vi "JPL Arm Control EX Autonomous.vi"(4 "Actual Angle":dbl, 5 "Arm Control":T1) -> (0 "Arm Status":T2, 3 "output":dbl)   [LabVIEW 2015]
panel:
  out "Arm Angle Chart":dbl(graph)
  out "PID Output Chart":dbl(graph)
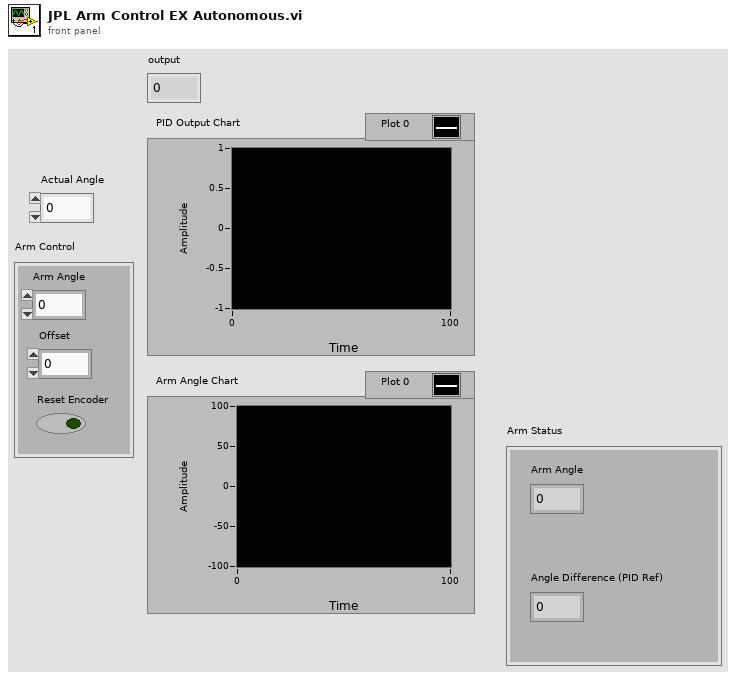
[diagram p1: front panel]
types:
  T1 = cluster{"Arm Angle":dbl, "Offset":dbl, "Reset Encoder":bool}
  T2 = cluster{"Arm Angle":dbl, "Angle Difference (PID Ref)":dbl}
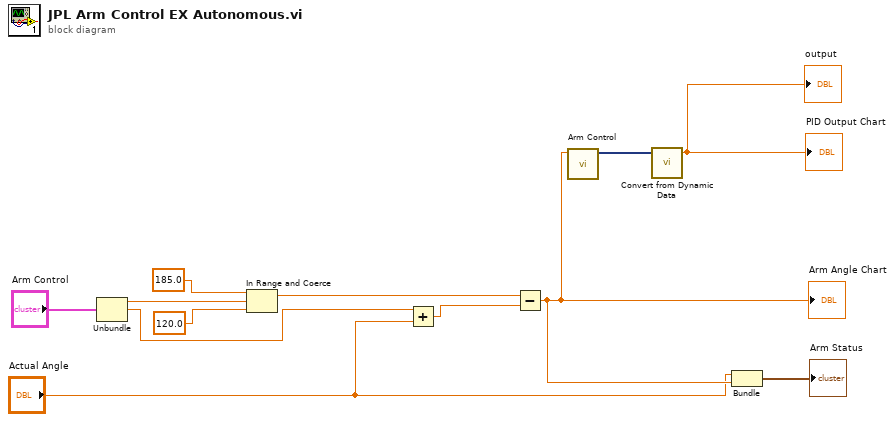
[diagram p0: block diagram]
diagram:
  n1 = Unbundle("Arm Control") -> ("Arm Angle"=w10:dbl, "Offset"=w2:dbl)  [unwired: 1 out]
  n2 = In Range and Coerce(upper limit=185.0, x=w10, lower limit=120.0) -> (coerced(x)=w7:dbl)  [unwired: 1 out]
  n3 = Add(x=w2, y="Actual Angle") -> (x+y=w1:dbl)
  n4 = Subtract(x=w7, y=w1) -> (x-y=w6:dbl)
  "Arm Angle Chart" <- w6
  n5 = call "Arm Control"("Signals"=w6) -> ("Scaled Signals"=w5:dynamicdata)  [unwired: 9 in, 1 out]
  n6 = call "Convert from Dynamic Data"("Dynamic Data Type"=w5) -> ("Scalar"=→"PID Output Chart" →"output":dbl)  [unwired: 3 in]
  n7 = Bundle("Actual Angle"="Actual Angle", w6) -> (→"Arm Status":cluster{"Actual Angle":dbl, dbl})  [unwired: 1 in]
